vi "AVQ8347 Center Peak.vi"(8 "Error In":errorcluster, 11 "VISA Session":refnum<visa-resource-name>) -> (0 "Error Out":errorcluster, 2 "Send Code":string, 3 "Copy VISA Session":refnum<visa-resource-name>)   [LabVIEW 2018]
doc: "To the center wavelength of the wavelength of the peak level setting"
panel:
  # "Center Peak"
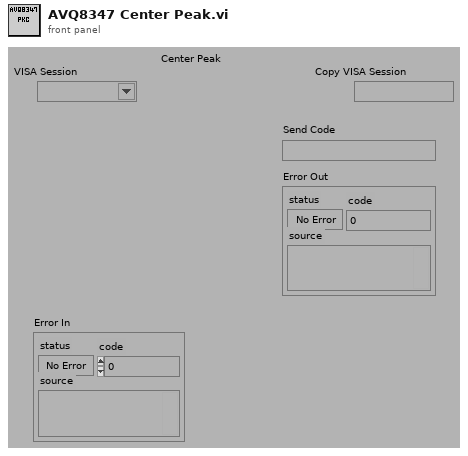
[diagram p1: front panel]
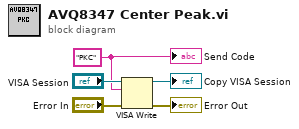
[diagram p0: block diagram]
diagram:
  w1 = "PKC"
  n1 = VISA Write(VISA resource name="VISA Session", write buffer=w1, error in (no error)="Error In") -> (VISA resource name out=→"Copy VISA Session":refnum<visa-resource-name>, error out=→"Error Out":errorcluster)  [unwired: 1 out]
  "Send Code" <- w1
